vi "Classification Particle Analysis.vi"(8 "error in (no error)":errorcluster, 10 "Image Dest":T1, 11 "Image Source":T1) -> (0 "error out":errorcluster, 1 "Center of Masses":cluster{"X":dbl, "Y":dbl}[](array[cluster]), 2 "ROIs":T2[](array[typedef]) {"Contours"."Type" items=["No Selection", "Point", "Line", "Rectangle", "Oval", "Polygon", "Freehand Region", "Annulus", "Unused2", "Unused3", "Broken Line", "Freehand Line", "Rotated Rectangle"]}, 3 "Image Out":T1)   [LabVIEW 2014]
doc: "This VI helps filter out unwanted particles and returns bounding box and center of mass information for the remaining particles."
uses:
  <vilib>/vision/Image Controls.llb/IMAQ Image.ctl
  <vilib>/vision/NI_Vision_Development_Module.lvlib
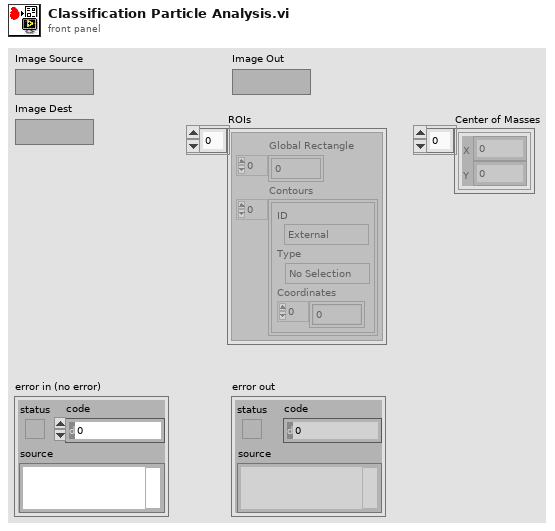
[diagram p1: front panel]
types:
  T1 = typedef "IMAQ Image.ctl" = refnum<image>
  T2 = typedef "ROI Descriptor" = cluster{"Global Rectangle":i32[], "Contours":cluster{"ID":enum32{"External", "Internal"}, "Type":u32, "Coordinates":i32[]}[]}
  T3 = cluster{"Area":dbl, "Number of Holes":dbl, "Bounding Rect":cluster{"Left":dbl, "Top":dbl, "Right":dbl, "Bottom":dbl}, "Center of Mass":cluster{"X":dbl, "Y":dbl}, "Orientation":dbl, "Dimensions":cluster{"Width":dbl, "Height":dbl}}[]
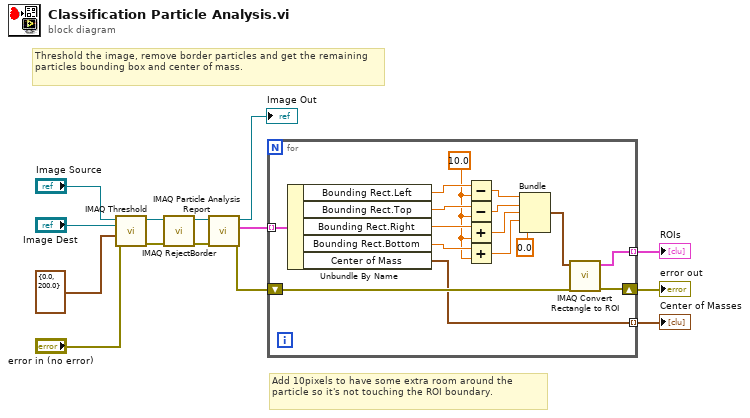
[diagram p0: block diagram]
diagram:
  # "Add 10pixels to have some extra room around the particle so it's not touching the ROI boundary."
  # "Threshold the image, remove border particles and get the remaining particles bounding box and center of mass."
  n1 = call "IMAQ Threshold"("error in (no error)"="error in (no error)", "Range"=cluster{"Lower value":sgl, "Upper value":sgl} {"Lower value"=0.0, "Upper value"=200.0}, "Image Dst"="Image Dest", "Image Src"="Image Source") -> ("error out"=w3:errorcluster, "Image Dst Out"=w4:T1)  [unwired: 2 in, 4 out]
  n2 = call "IMAQ RejectBorder"("error in (no error)"=w3, "Image Src"=w4) -> ("error out"=w1:errorcluster, "Image Dst Out"=w2:T1)  [unwired: 2 in, 2 out]
  n3 = call "IMAQ Particle Analysis Report"("error in (no error)"=w1, "Image"=w2) -> ("error out"=w10:errorcluster, "Particle Reports (Pixels)"=w12:T3, "Image Out (duplicate)"=→"Image Out":T1)  [unwired: 1 in, 6 out]
  n4 = for {
    tunnel: w12 -> [w30] mode=indexing
    tunnel: [w28] -> w11 mode=indexing
    shift-right: [w26] -> w9
    shift-left: w10 -> [w27]
    tunnel: [w25] -> w8 mode=indexing
    w17 = 10.0
    n5 = Unbundle By Name(w30) -> ("Bounding Rect.Left"=w24:dbl, "Bounding Rect.Top"=w23:dbl, "Bounding Rect.Right"=w20:dbl, "Bounding Rect.Bottom"=w19:dbl, "Center of Mass"=w25:cluster{"X":dbl, "Y":dbl})
    n6 = Subtract(x=w24, y=w17) -> (x-y=w22:dbl)
    n7 = Subtract(x=w23, y=w17) -> (x-y=w21:dbl)
    n8 = Add(x=w20, y=w17) -> (x+y=w15:dbl)
    n9 = Add(x=w19, y=w17) -> (x+y=w18:dbl)
    n10 = Bundle(w22, w21, w15, w18, 0.0) -> (w16:cluster{dbl, dbl, dbl, dbl, dbl})  [unwired: 1 out]
    n11 = call "IMAQ Convert Rectangle to ROI"("error in (no error)"=w27, "Rectangle"=w16) -> ("error out"=w26:errorcluster, "ROI Descriptor"=w28:T2)  [unwired: 7 out]
  }
  "ROIs" <- w11
  "error out" <- w9
  "Center of Masses" <- w8
